vi "h.SYSTEM.GetPowerCalibrationInfo.vi"(8 "error in":errorcluster, 11 "Connection ID":refnum<k5>) -> (0 "error out":errorcluster, 2 "power scales and offsets":i32[][](array[numeric]), 3 "Connection ID out":refnum<k5>)   [LabVIEW 2016, in "h.Library.lvlib"]
uses:
  h.Library.lvlib
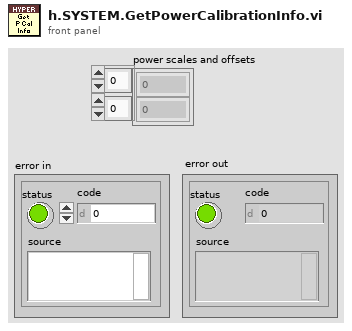
[diagram p1: front panel]
types:
  T1 = enum16{"big-endian, network order", "native, host order", "little-endian"}
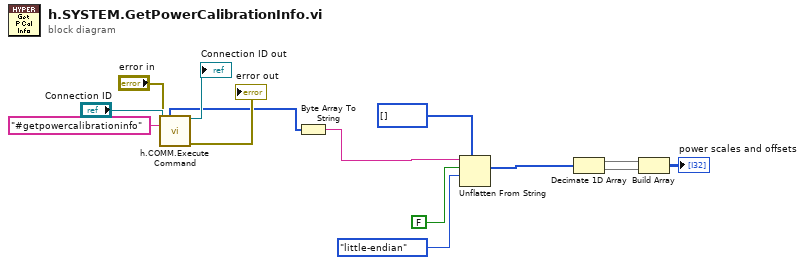
[diagram p0: block diagram]
diagram:
  n1 = call "h.COMM.Execute Command.vi"("Connection ID"="Connection ID", "Command"="#getpowercalibrationinfo", "error in"="error in") -> ("Content"=w1:u8[], "Connection ID out"=→"Connection ID out":refnum<k5>, "error out"=→"error out":errorcluster)  [unwired: 5 in, 5 out]
  n2 = Byte Array To String(unsigned byte array=w1) -> (string=w6:string)
  n3 = Unflatten From String(type=i32[] [], binary string=w6, data includes array or string size? (T)=FALSE, byte order (0:big-endian, network order)=T1."little-endian") -> (value=w5:i32[])  [unwired: 1 in, 2 out]
  n4 = Decimate 1D Array(w5) -> (w4:i32[], w3:i32[])
  n5 = Build Array(w4, w3) -> (→"power scales and offsets":i32[][])
